vi "Example_all-FINAL.vi"() -> ()   [LabVIEW 2020]
uses:
  <vilib>/httpClient/MultipartData.ctl
  <vilib>/httpClient/POSTBuffer.vi
  <vilib>/httpClient/LabVIEWHTTPClient.lvlib
panel:
  out "status":string
  out "Config":string
  out "Test Bench List":string
  in  "Path":path
  out "Version":string
  in  "parameter":i16=1
  in  "contrast":dbl=0.02
  in  "edge":i16=10
  in  "subcell":i16=101
  in  "filtertype":string(combo)="gaussian"
  in  "test bench identifier":string="test"
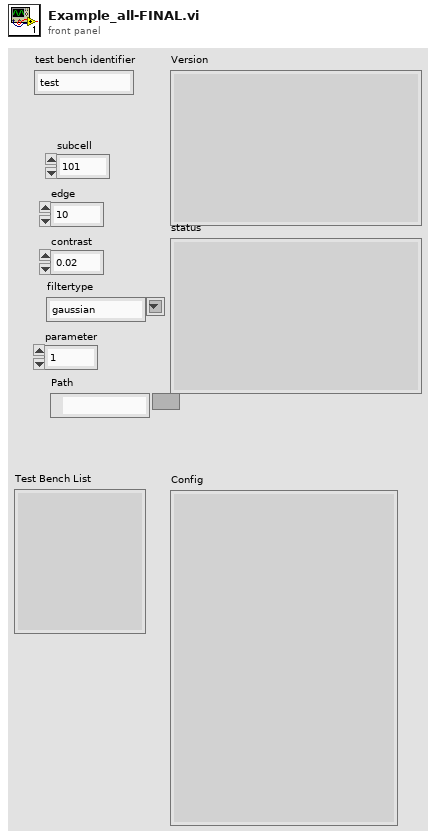
[diagram p1: front panel]
types:
  T1 = typedef "LabVIEWHTTPClient.lvlib/MultipartData.ctl" = cluster{"Name":string, "Value":string, "File":path, "Filename":string, "MIME type":string}
  T2 = typedef "LabVIEWHTTPClient.lvlib/ClientHandle.ctl" = refnum<k1>
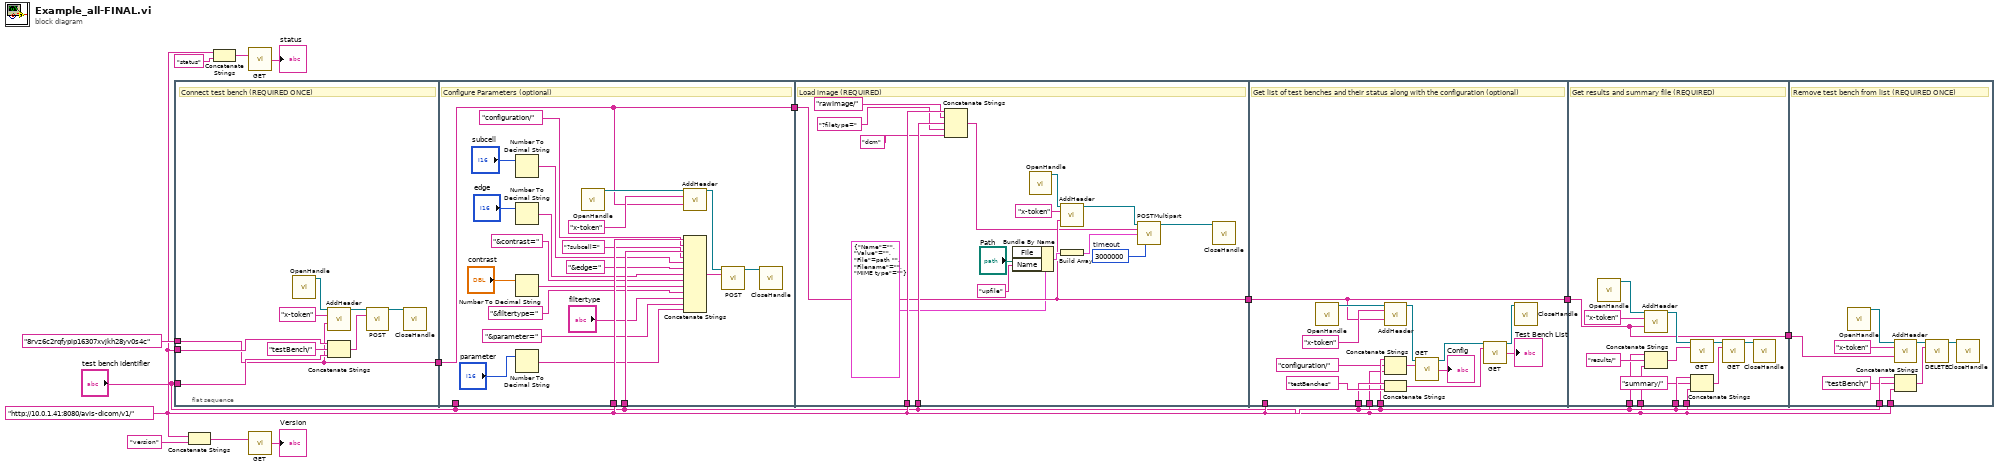
[diagram p0: block diagram]
diagram:
  w3 = "http://10.0.1.41:8080/avis-dicom/v1/"
  n1 = flat-sequence {
    tunnel: w3 -> [w21]
    tunnel: "test bench identifier" -> [w20]
    tunnel: "8rvz6c2rqfypip16307xvjkh28yv0s4c" -> [w15]
    tunnel: [w15] -> w10
    tunnel: w3 -> [w46]
    tunnel: "test bench identifier" -> [_]
    tunnel: "test bench identifier" -> [w44]
    tunnel: w10 -> [w24]
    tunnel: [w24] -> w9
    tunnel: w3 -> [w63]
    tunnel: "test bench identifier" -> [w61]
    tunnel: [w55] -> w1
    tunnel: w9 -> [w55]
    tunnel: w3 -> [_]
    tunnel: w3 -> [w76]
    tunnel: w1 -> [w68]
    tunnel: [w68] -> w8
    tunnel: w3 -> [w67]
    tunnel: "test bench identifier" -> [w65]
    tunnel: w3 -> [w89]
    tunnel: w3 -> [w88]
    tunnel: "test bench identifier" -> [w86]
    tunnel: "test bench identifier" -> [w85]
    tunnel: w8 -> [w79]
    tunnel: [w79] -> w7
    tunnel: w3 -> [w100]
    tunnel: "test bench identifier" -> [w98]
    tunnel: w7 -> [w97]
    frame #0 {
      # "Connect test bench (REQUIRED ONCE)"
      n2 = call <vilib>:"OpenHandle.vi"() -> ("client handle out"=w18:T2)  [unwired: 14 in, 1 out]
      n3 = call <vilib>:"AddHeader.vi"("client handle"=w18, "header"="x-token", "value"=w15) -> ("client handle out"=w17:T2)  [unwired: 11 in, 1 out]
      n4 = Concatenate Strings(w21, "testBench/", w20) -> (w23:string)
      n5 = call-poly <vilib>:"POST.vi"("client handle"=w17, "url"=w23) -> ("client handle out"=w16:T2)  [unwired: 10 in, 3 out]
      n6 = call <vilib>:"CloseHandle.vi"("client handle"=w16) -> ()  [unwired: 14 in, 1 out]
    }
    frame #1 {
      # "Configure Parameters (optional)"
      n7 = Number To Decimal String(number="subcell") -> (decimal integer string=w41:string)  [unwired: 1 in]
      n8 = Number To Decimal String(number="edge") -> (decimal integer string=w38:string)  [unwired: 1 in]
      n9 = Number To Decimal String(number="contrast") -> (decimal integer string=w35:string)  [unwired: 1 in]
      n10 = Number To Decimal String(number="parameter") -> (decimal integer string=w30:string)  [unwired: 1 in]
      n11 = call <vilib>:"OpenHandle.vi"() -> ("client handle out"=w28:T2)  [unwired: 14 in, 1 out]
      n12 = call <vilib>:"AddHeader.vi"("client handle"=w28, "header"="x-token", "value"=w24) -> ("client handle out"=w27:T2)  [unwired: 11 in, 1 out]
      n13 = Concatenate Strings(w46, "configuration/", w44, "?subcell=", w41, "&edge=", w38, "&contrast=", w35, "&filtertype=", "filtertype", "&parameter=", w30) -> (w29:string)
      n14 = call-poly <vilib>:"POST.vi"("client handle"=w27, "url"=w29) -> ("client handle out"=w26:T2)  [unwired: 10 in, 3 out]
      n15 = call <vilib>:"CloseHandle.vi"("client handle"=w26) -> ()  [unwired: 14 in, 1 out]
    }
    frame #2 {
      w52 = 3000000  # timeout
      # "Load image (REQUIRED)"
      n16 = Concatenate Strings(w63, "rawImage/", w61, "?filetype=", "dcm") -> (w50:string)
      n17 = Bundle By Name(cluster=T1 {"Name"="", "Value"="", "File"=path "", "Filename"="", "MIME type"=""} ("Element"), "File"="Path", "Name"="upfile") -> (w58:T1)
      n18 = call <vilib>:"OpenHandle.vi"() -> ("client handle out"=w57:T2)  [unwired: 14 in, 1 out]
      n19 = call <vilib>:"AddHeader.vi"("client handle"=w57, "header"="x-token", "value"=w55) -> ("client handle out"=w54:T2)  [unwired: 11 in, 1 out]
      n20 = Build Array(w58) -> (w51:T1[])
      n21 = call <vilib>:"POSTMultipart.vi"("client handle"=w54, "url"=w50, "data"=w51, "timeout (10000)"=w52) -> ("client handle out"=w53:T2)  [unwired: 8 in, 3 out]
      n22 = call <vilib>:"CloseHandle.vi"("client handle"=w53) -> ()  [unwired: 14 in, 1 out]
    }
    frame #3 {
      # "Get list of test benches and their status along with the configuration (optional)"
      n23 = call <vilib>:"OpenHandle.vi"() -> ("client handle out"=w72:T2)  [unwired: 14 in, 1 out]
      n24 = call <vilib>:"AddHeader.vi"("client handle"=w72, "header"="x-token", "value"=w68) -> ("client handle out"=w73:T2)  [unwired: 11 in, 1 out]
      n25 = Concatenate Strings(w67, "configuration/", w65) -> (w70:string)
      n26 = Concatenate Strings(w76, "testBenches") -> (w75:string)
      n27 = call <vilib>:"GET.vi"("client handle"=w73, "url"=w70) -> ("client handle out"=w64:T2, "body"=→"Config":string)  [unwired: 10 in, 2 out]
      n28 = call <vilib>:"GET.vi"("client handle"=w64, "url"=w75) -> ("client handle out"=w74:T2, "body"=→"Test Bench List":string)  [unwired: 10 in, 2 out]
      n29 = call <vilib>:"CloseHandle.vi"("client handle"=w74) -> ()  [unwired: 14 in, 1 out]
    }
    frame #4 {
      # "Get results and summary file (REQUIRED)"
      n30 = call <vilib>:"OpenHandle.vi"() -> ("client handle out"=w83:T2)  [unwired: 14 in, 1 out]
      n31 = call <vilib>:"AddHeader.vi"("client handle"=w83, "header"="x-token", "value"=w79) -> ("client handle out"=w82:T2)  [unwired: 11 in, 1 out]
      n32 = Concatenate Strings(w89, "results/", w85) -> (w92:string)
      n33 = call <vilib>:"GET.vi"("client handle"=w82, "url"=w92) -> ("client handle out"=w81:T2)  [unwired: 10 in, 3 out]
      n34 = Concatenate Strings(w88, "summary/", w86) -> (w91:string)
      n35 = call <vilib>:"GET.vi"("client handle"=w81, "url"=w91) -> ("client handle out"=w80:T2)  [unwired: 10 in, 3 out]
      n36 = call <vilib>:"CloseHandle.vi"("client handle"=w80) -> ()  [unwired: 14 in, 1 out]
    }
    frame #5 {
      # "Remove test bench from list (REQUIRED ONCE)"
      n37 = call <vilib>:"OpenHandle.vi"() -> ("client handle out"=w95:T2)  [unwired: 14 in, 1 out]
      n38 = call <vilib>:"AddHeader.vi"("client handle"=w95, "header"="x-token", "value"=w97) -> ("client handle out"=w94:T2)  [unwired: 11 in, 1 out]
      n39 = Concatenate Strings(w100, "testBench/", w98) -> (w101:string)
      n40 = call <vilib>:"DELETE.vi"("client handle"=w94, "url"=w101) -> ("client handle out"=w93:T2)  [unwired: 10 in, 3 out]
      n41 = call <vilib>:"CloseHandle.vi"("client handle"=w93) -> ()  [unwired: 14 in, 1 out]
    }
  }
  n42 = Concatenate Strings(w3, "version") -> (w13:string)
  n43 = Concatenate Strings(w3, "status") -> (w6:string)
  n44 = call <vilib>:"GET.vi"("url"=w6) -> ("body"=→"status":string)  [unwired: 11 in, 3 out]
  n45 = call <vilib>:"GET.vi"("url"=w13) -> ("body"=→"Version":string)  [unwired: 11 in, 3 out]
